vi "GV C00.vi"() -> ()   [LabVIEW 2017]
panel:
  in  "C00":u8
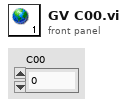
[diagram p1: front panel]
diagram:
